vi "run.vi"(8 "error in (no error)":errorcluster, 11 "SettingsManager in":refnum<class "SettingsManager.lvclass">) -> (0 "error out":errorcluster, 3 "SettingsManager out":refnum<class "SettingsManager.lvclass">)   [LabVIEW 2011, in "Tools.lvlib" / "Settings.lvlib" / "SettingsManager.lvclass"]
uses:
  SettingsManager.lvclass
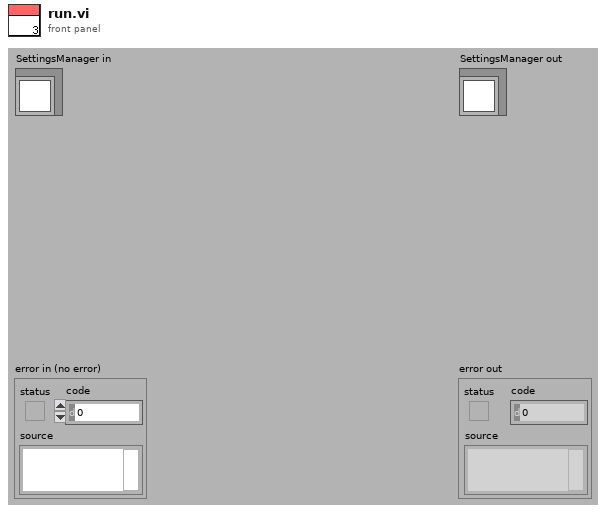
[diagram p1: front panel]
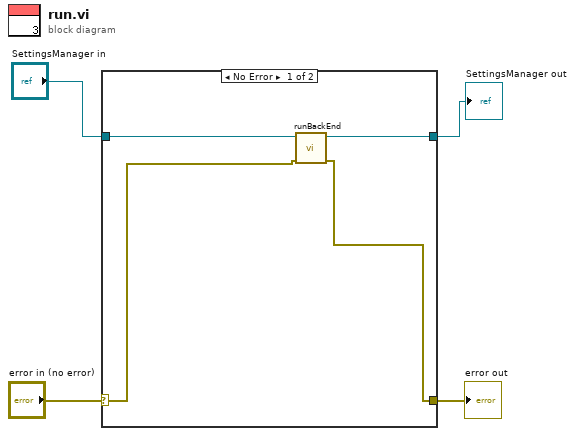
[diagram p0: block diagram]
diagram:
  n1 = case shown="No Error" "error in (no error)" {
    selector: "error in (no error)" -> [w6 w10]
    tunnel: [w5 w10] -> w3
    tunnel: [w8 w9] -> w1
    tunnel: "SettingsManager in" -> [w7 w9]
    frame No Error {
      n2 = call "runBackEnd.vi"("error in (no error)"=w6, "SettingsManager in"=w7) -> ("error out"=w5:errorcluster, "SettingsManager out"=w8:refnum<class "SettingsManager.lvclass">)  [unwired: 8 in]
    }
    frame Error {
    }
  }
  "error out" <- w3
  "SettingsManager out" <- w1
